vi "Lab1_Exercise1.vi"() -> ()   [LabVIEW 2016]
panel:
  out "Gauge":dbl(knob) scale=0.0..60.0
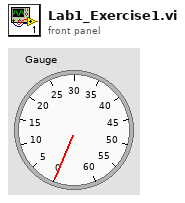
[diagram p1: front panel]
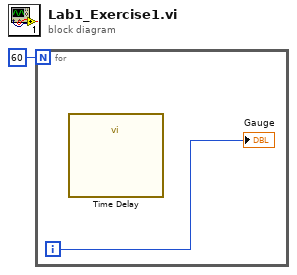
[diagram p0: block diagram]
diagram:
  n1 = for {
    N: 60 -> [_]
    i -> [w2]
    n2 = call "Time Delay"() -> ()  [unwired: 11 in, 1 out]
    "Gauge" <- w2
  }
